vi "Zyklussteuerung.vi"(0 "FPGA VI Reference In":refnum<k20>, 1 "DIOsNummern":cluster{"DIOsMod2BNr":i32[]}[](array[cluster]), 2 "Zyklusnummern 0, 1, 2A, 2B":i32[](array[numeric]), 3 "Zykluszeiten 0, 1, 2A, 2B":dbl[](array[numeric]), 4 "Zeitpkte/SPs":T1 {"FPGAPID"."proportional gain (Kc)" format="%.11g"; "FPGAPID"."integral gain (Kc*Ts/Ti)" format="%.11g"; "FPGAPID"."derivative gain (Kc*Td/Ts)" format="%.11g"; "FPGAFixp" format="%.14g"}, 5 "HorstSP":dbl[](array[numeric]), 6 "ZwangsDIO?":cluster{bool[]}[](array[cluster]), 7 "ZwangsLangsameH?":bool[](array[boolean]), 8 "ZwangsDIO!":cluster{bool[]}[](array[cluster]), 9 "ZwangsLangsameH!":bool[](array[boolean]), 10 "ZwangsHorst?":cluster{bool[]}[](array[cluster]), 11 "ZwangsFPGABoolesch?":bool[](array[boolean]), 12 "ZwangsHorst!":cluster{dbl[]}[](array[cluster]), 13 "ZwangsFPGABoolesch!":bool[](array[boolean]), 14 "Schieberegister":T2) -> (15 "HorstSP":dbl[](array[numeric]), 17 "Heizen?LH":bool[](array[boolean]), 19 "Schieberegister":T2)   [LabVIEW 2010]
uses:
  <vilib>/rvi/interface/nirviReadWriteControl/nirviReadWriteControl.xnode
  C:/Users/HAGAR-IV/Desktop/Zeugs/markus/version feb 2012/FPGA Bitfiles/pertrasgcfpga2_FPGATarget_FPGA-Programm-10_16368CB6.lvbitx
  C:/Users/HAGAR-IV/Desktop/Zeugs/Johnny/pertrasgc fpga/FPGA-Programm-10-14.vi
  <vilib>/rvi/interface/common/niFpgaNodeNameForErrorReporting.ctl
  <vilib>/rvi/errors/niLvFpgaWhatHappensToTopLevelVI.ctl
  <vilib>/Utility/error.llb/Error Cluster From Error Code.vi
  <vilib>/rvi/errors/niLvFpgaAdjustHostInterfaceError.vi
  NiFpgaLv.dll
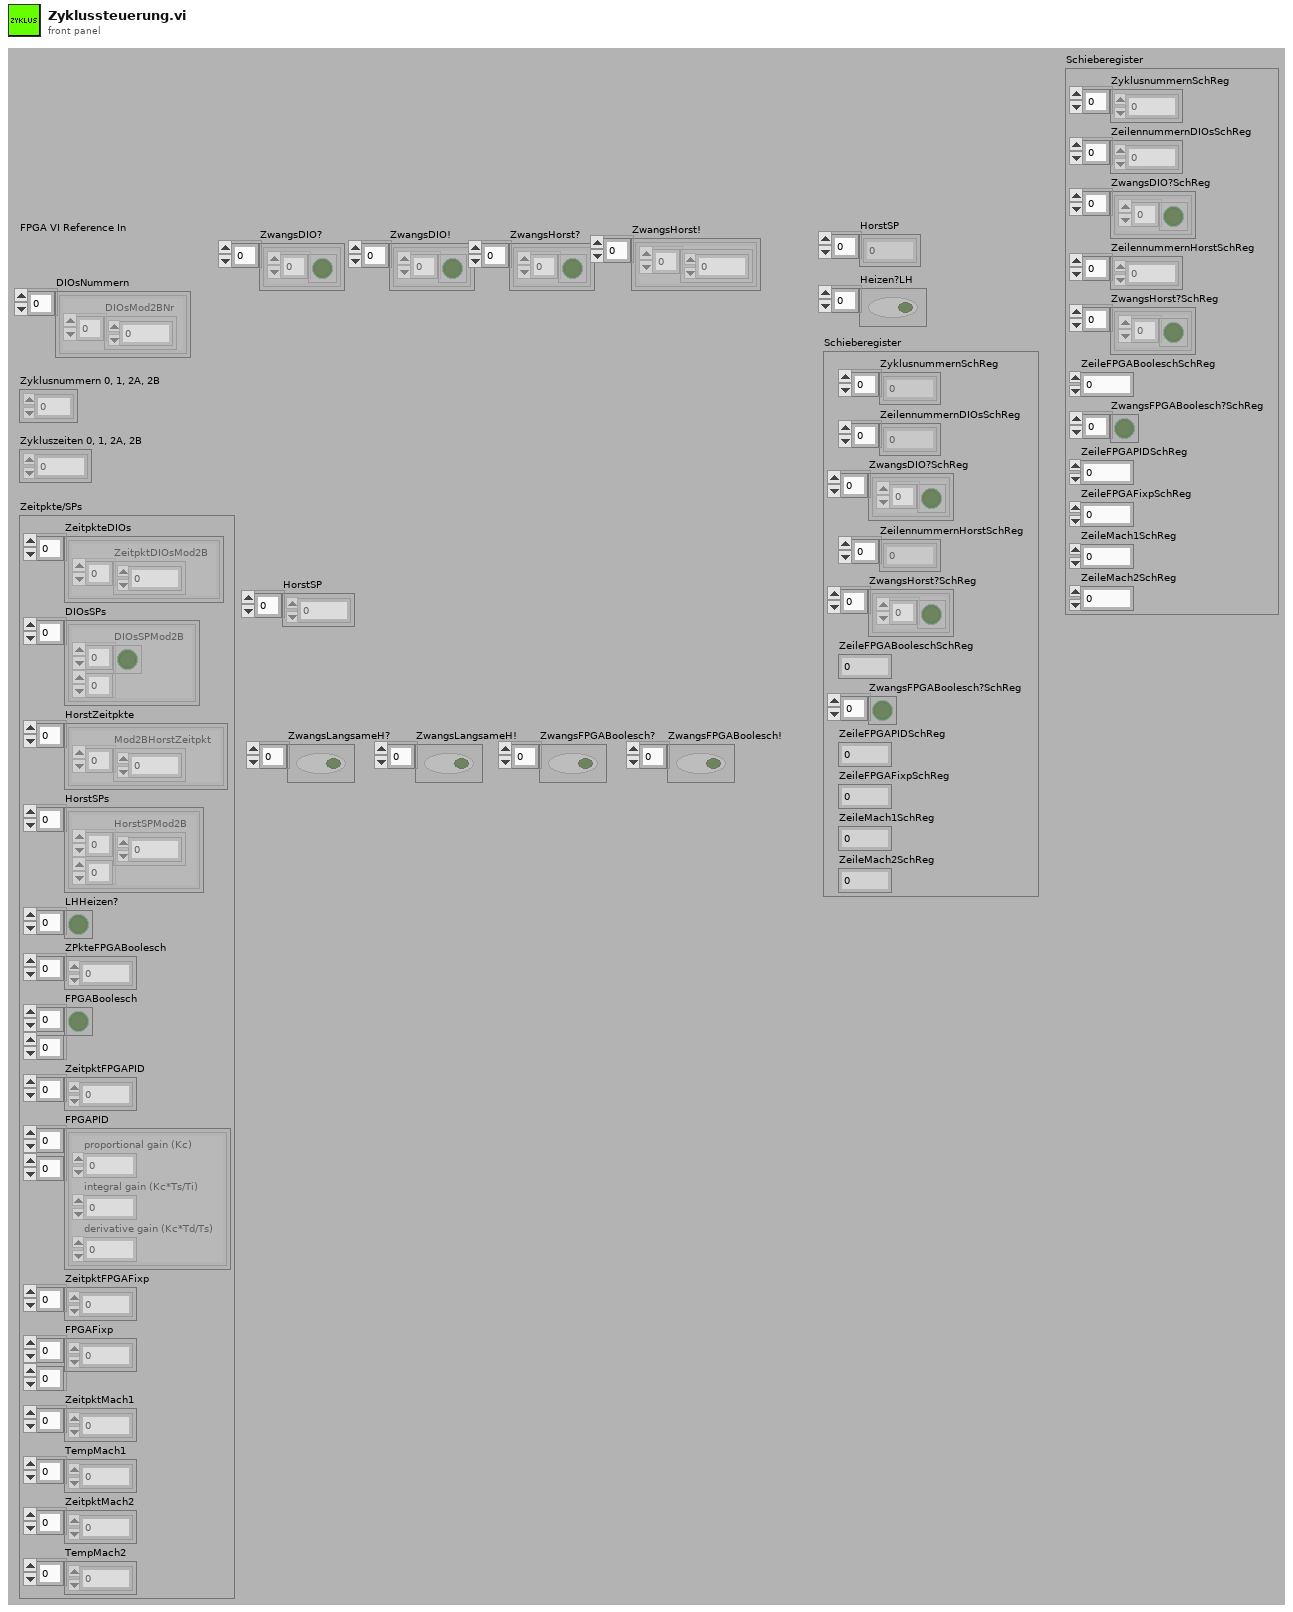
[diagram p1: front panel]
types:
  T1 = cluster{"ZeitpkteDIOs":cluster{"ZeitpktDIOsMod2B":dbl[]}[], "DIOsSPs":cluster{"DIOsSPMod2B":bool[][]}[], "HorstZeitpkte":cluster{"Mod2BHorstZeitpkt":dbl[]}[], "HorstSPs":cluster{"HorstSPMod2B":dbl[][]}[], "LHHeizen?":bool[], "ZPkteFPGABoolesch":dbl[], "FPGABoolesch":bool[][], "ZeitpktFPGAPID":dbl[], "FPGAPID":cluster{"proportional gain (Kc)":fxp<+/-,16,8>, "integral gain (Kc*Ts/Ti)":fxp<+/-,16,8>, "derivative gain (Kc*Td/Ts)":fxp<+/-,16,8>}[][], "ZeitpktFPGAFixp":dbl[], "FPGAFixp":fxp<+/-,16,4>[][], "ZeitpktMach1":dbl[], "TempMach1":dbl[], "ZeitpktMach2":dbl[], "TempMach2":dbl[]}
  T2 = cluster{"ZyklusnummernSchReg":i32[], "ZeilennummernDIOsSchReg":i32[], "ZwangsDIO?SchReg":cluster{bool[]}[], "ZeilennummernHorstSchReg":i32[], "ZwangsHorst?SchReg":cluster{bool[]}[], "ZeileFPGABooleschSchReg":i32, "ZwangsFPGABoolesch?SchReg":bool[], "ZeileFPGAPIDSchReg":i32, "ZeileFPGAFixpSchReg":i32, "ZeileMach1SchReg":i32, "ZeileMach2SchReg":i32}
  T3 = cluster{"proportional gain (Kc)":fxp<+/-,16,8>, "integral gain (Kc*Ts/Ti)":fxp<+/-,16,8>, "derivative gain (Kc*Td/Ts)":fxp<+/-,16,8>}[][]
  T4 = typedef "niFpgaNodeNameForErrorReporting.ctl" = enum16{"Open FPGA VI Reference", "Read/Write Control", "Invoke Method: Abort", "Invoke Method: Acknowledge IRQ", "Invoke Method: Download", "Invoke Method: FIFO.Configure", "Invoke Method: FIFO.Read", "Invoke Method: FIFO.Start", "Invoke Method: FIFO.Stop", "Invoke Method: FIFO.Write", "Invoke Method: Reset", "Invoke Method: Run", "Invoke Method: Wait on IRQ", "Close FPGA VI Reference"}
  T5 = typedef "niLvFpgaWhatHappensToTopLevelVI.ctl" = enum16{"top level VI scripted behind XNode", "top level VI inlined behind XNode"}
  T6 = cluster{"FPGAFixp[0]":fxp<+/-,16,4>, "FPGAFixp[1]":fxp<+/-,16,4>, "FPGAFixp[2]":fxp<+/-,16,4>, "FPGAFixp[3]":fxp<+/-,16,4>, "FPGAFixp[4]":fxp<+/-,16,4>, "FPGAFixp[5]":fxp<+/-,16,4>, "FPGAFixp[6]":fxp<+/-,16,4>, "FPGAFixp[7]":fxp<+/-,16,4>}
  T7 = cluster{"proportional gain (Kc)":fxp<+/-,16,8>, "integral gain (Kc*Ts/Ti)":fxp<+/-,16,8>, "derivative gain (Kc*Td/Ts)":fxp<+/-,16,8>}[]
  T8 = cluster{"FPGAPID[0]":cluster{"proportional gain (Kc)":fxp<+/-,16,8>, "integral gain (Kc*Ts/Ti)":fxp<+/-,16,8>, "derivative gain (Kc*Td/Ts)":fxp<+/-,16,8>}, "FPGAPID[1]":cluster{"proportional gain (Kc)":fxp<+/-,16,8>, "integral gain (Kc*Ts/Ti)":fxp<+/-,16,8>, "derivative gain (Kc*Td/Ts)":fxp<+/-,16,8>}, "FPGAPID[2]":cluster{"proportional gain (Kc)":fxp<+/-,16,8>, "integral gain (Kc*Ts/Ti)":fxp<+/-,16,8>, "derivative gain (Kc*Td/Ts)":fxp<+/-,16,8>}, "FPGAPID[3]":cluster{"proportional gain (Kc)":fxp<+/-,16,8>, "integral gain (Kc*Ts/Ti)":fxp<+/-,16,8>, "derivative gain (Kc*Td/Ts)":fxp<+/-,16,8>}}
  T9 = cluster{"proportional gain (Kc)":fxp<+/-,16,8>, "integral gain (Kc*Ts/Ti)":fxp<+/-,16,8>, "derivative gain (Kc*Td/Ts)":fxp<+/-,16,8>}
  T10 = cluster{"[0]":bool, "[1]":bool, "[2]":bool, "[3]":bool, "[4]":bool, "[5]":bool}
  T11 = cluster{"[0]":bool, "[1]":bool, "[2]":bool, "[3]":bool, "[4]":bool, "[5]":bool, "[6]":bool, "[7]":bool, "[8]":bool, "[9]":bool, "[10]":bool, "[11]":bool, "[12]":bool, "[13]":bool, "[14]":bool, "[15]":bool, "[16]":bool, "[17]":bool, "[18]":bool, "[19]":bool, "[20]":bool, "[21]":bool, "[22]":bool, "[23]":bool, "[24]":bool, "[25]":bool, "[26]":bool, "[27]":bool, "[28]":bool, "[29]":bool, "[30]":bool, "[31]":bool}
  T12 = cluster{"Zyklusnummern 0, 1, 2A, 2B":i32[], i32[], "ZwangsDIO?":cluster{bool[]}[], i32[], "ZwangsHorst?":cluster{bool[]}[], i32, "ZwangsFPGABoolesch?":bool[], i32, i32, i32, i32}
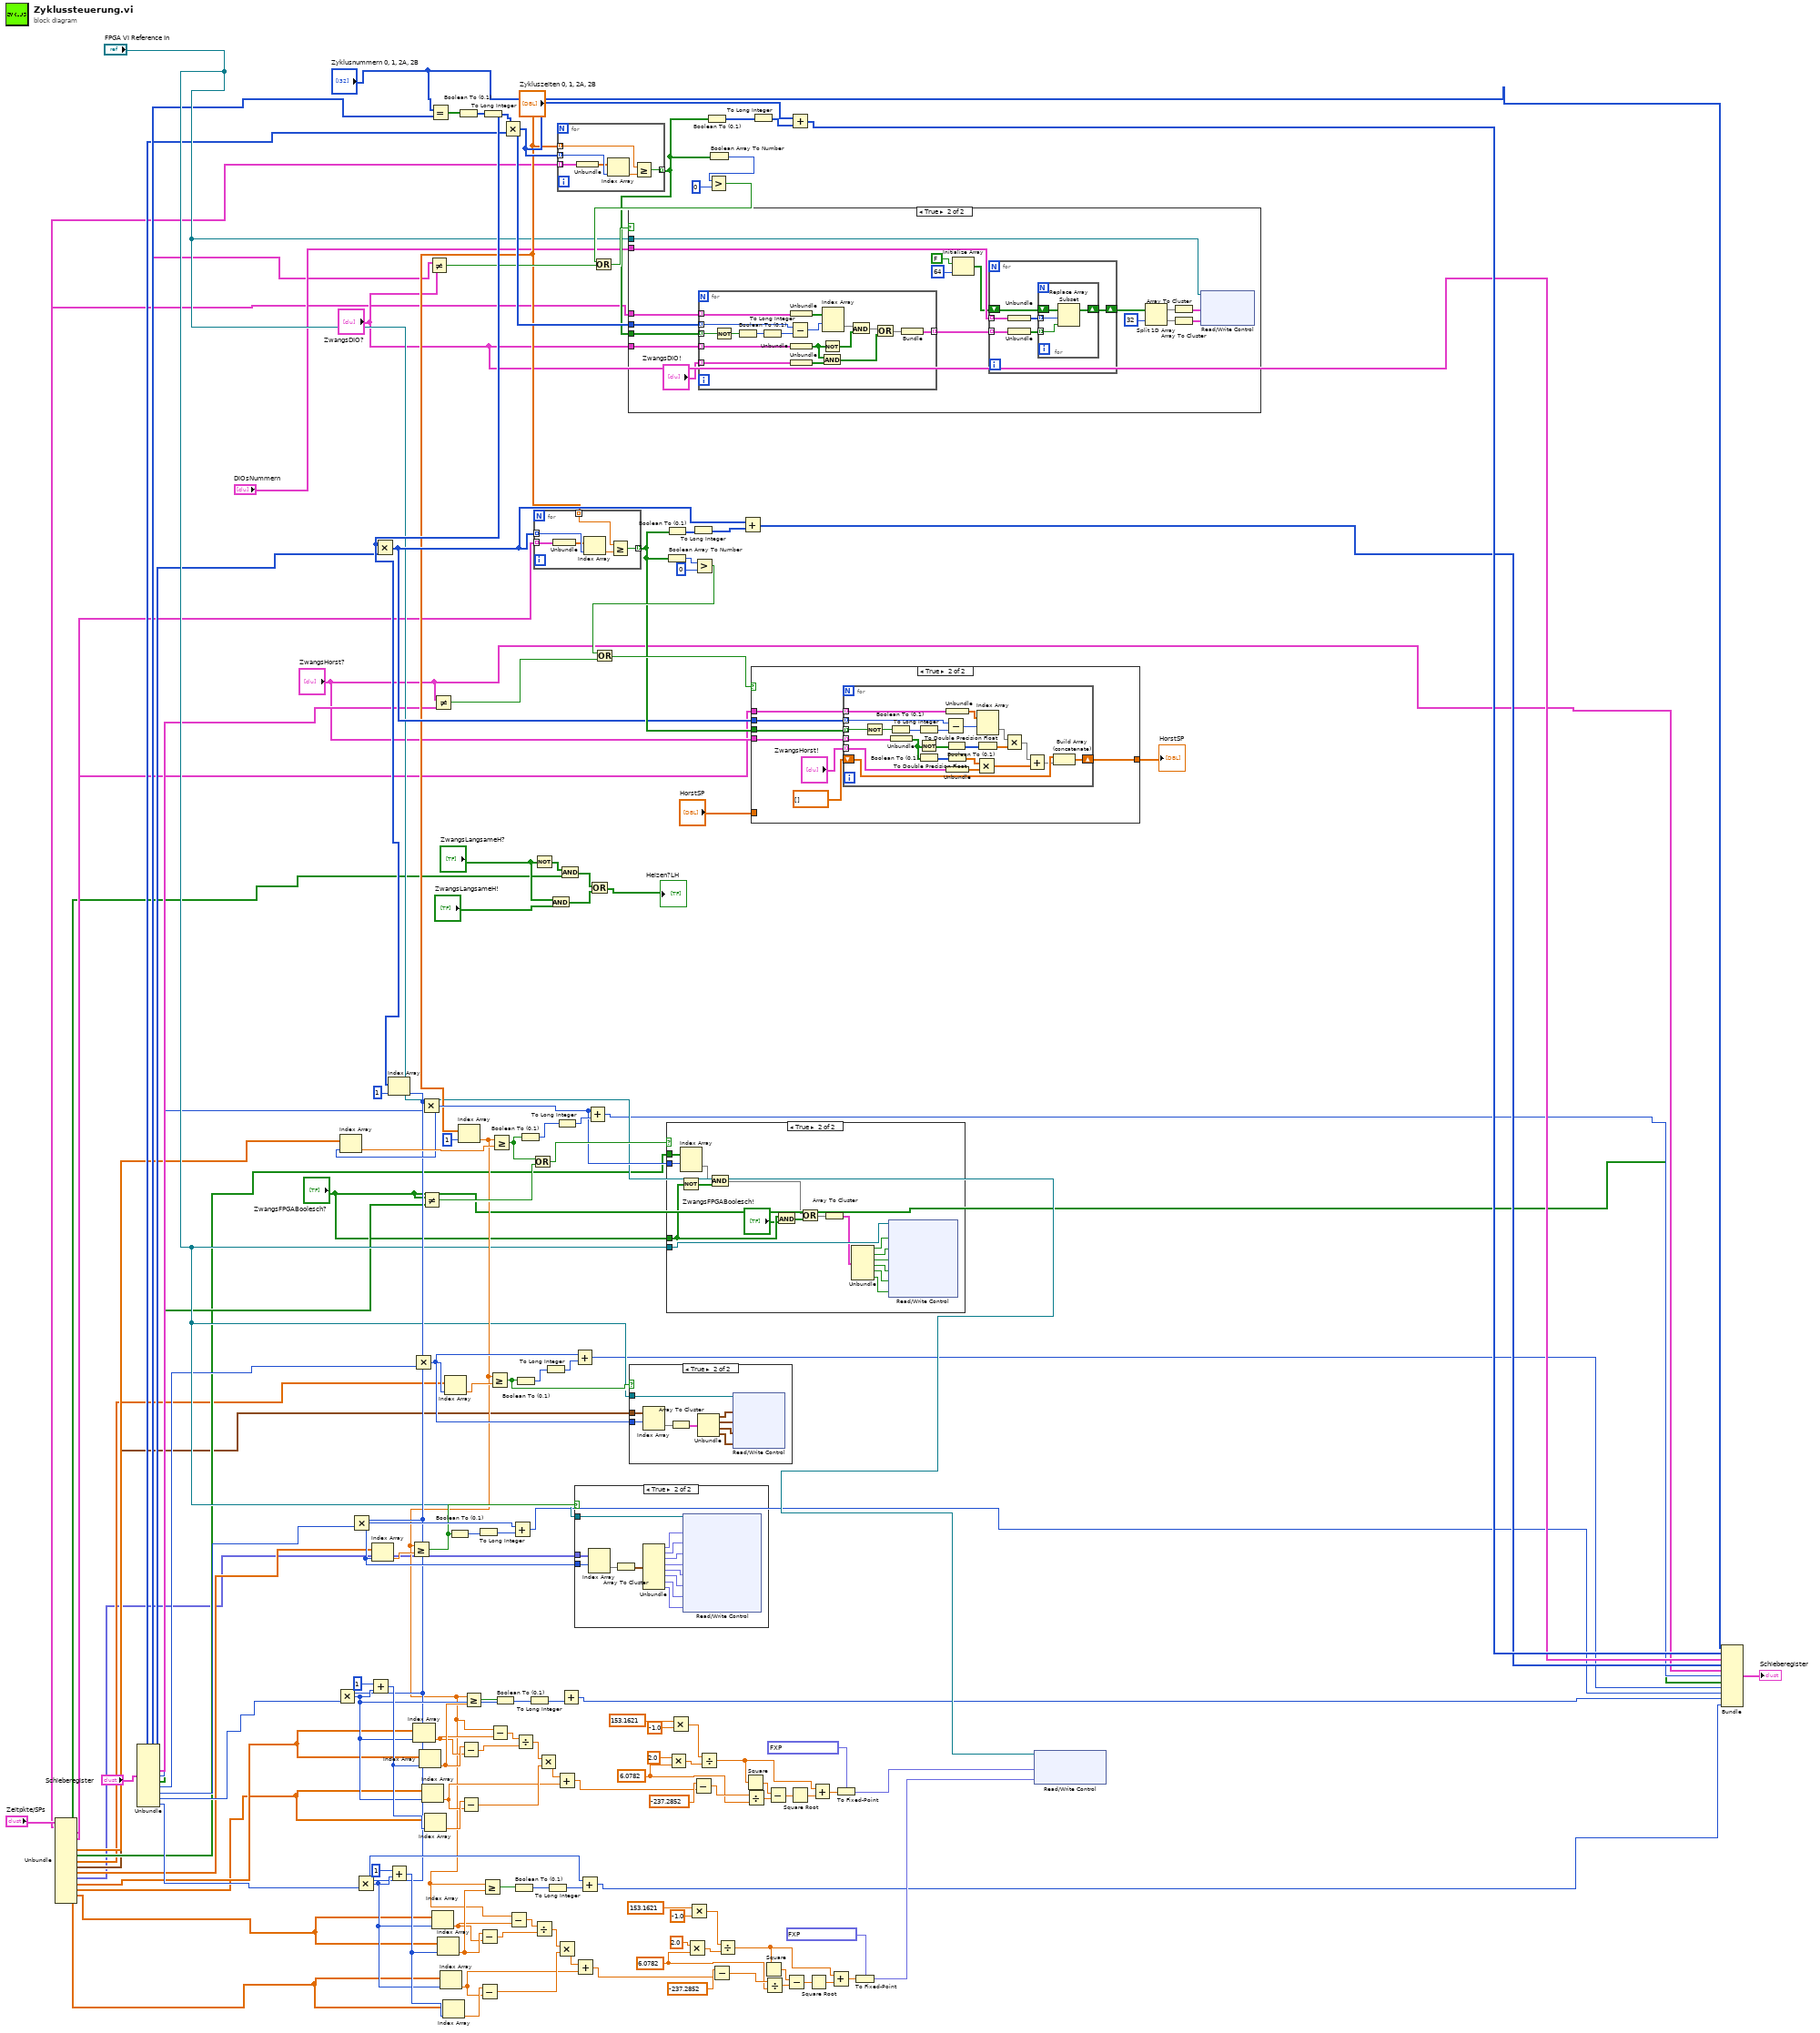
[diagram p0: block diagram]
diagram:
  w67 = 6.0782 ("y")
  w99 = 6.0782 ("y")
  n1 = Unbundle("Zeitpkte/SPs") -> ("ZeitpkteDIOs"=w17:cluster{"ZeitpktDIOsMod2B":dbl[]}[], "DIOsSPs"=w16:cluster{"DIOsSPMod2B":bool[][]}[], "HorstZeitpkte"=w15:cluster{"Mod2BHorstZeitpkt":dbl[]}[], "HorstSPs"=w14:cluster{"HorstSPMod2B":dbl[][]}[], "LHHeizen?"=w13:bool[], "ZPkteFPGABoolesch"=w12:dbl[], "FPGABoolesch"=w11:bool[][], "ZeitpktFPGAPID"=w10:dbl[], "FPGAPID"=w9:T3, "ZeitpktFPGAFixp"=w8:dbl[], "FPGAFixp"=w7:fxp<+/-,16,4>[][], "ZeitpktMach1"=w6:dbl[], "TempMach1"=w5:dbl[], "ZeitpktMach2"=w4:dbl[], "TempMach2"=w3:dbl[])
  n2 = Unbundle("Schieberegister") -> ("ZyklusnummernSchReg"=w41:i32[], "ZeilennummernDIOsSchReg"=w40:i32[], "ZwangsDIO?SchReg"=w39:cluster{bool[]}[], "ZeilennummernHorstSchReg"=w38:i32[], "ZwangsHorst?SchReg"=w37:cluster{bool[]}[], "ZeileFPGABooleschSchReg"=w36:i32, "ZwangsFPGABoolesch?SchReg"=w35:bool[], "ZeileFPGAPIDSchReg"=w34:i32, "ZeileFPGAFixpSchReg"=w33:i32, "ZeileMach1SchReg"=w32:i32, "ZeileMach2SchReg"=w31:i32)
  n3 = Not Equal?(x="ZwangsFPGABoolesch?", y=w35) -> (x != y?=w137:bool)
  n4 = Not Equal?(x=w39, y="ZwangsDIO?") -> (x != y?=w51:bool)
  n5 = Equal?(x="Zyklusnummern 0, 1, 2A, 2B", y=w41) -> (x = y?=w157:bool[])
  n6 = Not Equal?(x="ZwangsHorst?", y=w37) -> (x != y?=w52:bool)
  n7 = Boolean To (0,1)(Boolean=w157) -> (0, 1=w156:i16[])
  n8 = Index Array(array="Zykluszeiten 0, 1, 2A, 2B", index=1 ("Index")) -> (element=w63:dbl)
  n9 = To Long Integer(number=w156) -> (32bit integer=w144:i32[])
  n10 = Multiply(x=w144, y=w38) -> (x*y=w53:i32[])
  n11 = Index Array(array=w144, index=1 ("Index")) -> (element=w64:i32)
  n12 = Multiply(x=w64, y=w32) -> (x*y=w117:i32)
  n13 = Multiply(x=w64, y=w33) -> (x*y=w126:i32)
  n14 = Multiply(x=w64, y=w31) -> (x*y=w87:i32)
  n15 = Add(x=1 ("y"), y=w117) -> (x+y=w123:i32)
  n16 = Index Array(array=w8, index=w126) -> (element=w129:dbl)
  n17 = Add(x=1 ("y"), y=w87) -> (x+y=w93:i32)
  n18 = Greater Or Equal?(x=w63, y=w129) -> (x >= y?=w125:bool)
  n19 = Multiply(x=w64, y=w34) -> (x*y=w130:i32)
  n20 = Index Array(array=w6, index=w117) -> (element=w116:dbl)
  n21 = Index Array(array=w6, index=w123) -> (element=w121:dbl)
  n22 = Multiply(x=w64, y=w36) -> (x*y=w135:i32)
  n23 = Index Array(array=w12, index=w135) -> (element=w141:dbl)
  n24 = Index Array(array=w5, index=w117) -> (element=w110:dbl)
  n25 = Index Array(array=w5, index=w123) -> (element=w122:dbl)
  n26 = Index Array(array=w4, index=w87) -> (element=w86:dbl)
  n27 = Index Array(array=w4, index=w93) -> (element=w91:dbl)
  n28 = Index Array(array=w3, index=w87) -> (element=w80:dbl)
  n29 = Index Array(array=w3, index=w93) -> (element=w92:dbl)
  n30 = Index Array(array=w10, index=w130) -> (element=w134:dbl)
  n31 = Boolean To (0,1)(Boolean=w125) -> (0, 1=w128:i16)
  n32 = Subtract(x=w121, y=w116) -> (x-y=w114:dbl)
  n33 = Subtract(x=w122, y=w110) -> (x-y=w112:dbl)
  n34 = Greater Or Equal?(x=w63, y=w121) -> (x >= y?=w120:bool)
  n35 = To Long Integer(number=w128) -> (32bit integer=w127:i32)
  n36 = Subtract(x=w91, y=w86) -> (x-y=w84:dbl)
  n37 = Subtract(x=w92, y=w80) -> (x-y=w82:dbl)
  n38 = Greater Or Equal?(x=w63, y=w91) -> (x >= y?=w90:bool)
  n39 = Greater Or Equal?(x=w63, y=w134) -> (x >= y?=w131:bool)
  n40 = Subtract(x=w63, y=w116) -> (x-y=w115:dbl)
  n41 = Greater Or Equal?(x=w63, y=w141) -> (x >= y?=w138:bool)
  n42 = Boolean To (0,1)(Boolean=w120) -> (0, 1=w119:i16)
  n43 = Multiply(x=w144, y=w40) -> (x*y=w56:i32[])
  n44 = Subtract(x=w63, y=w86) -> (x-y=w85:dbl)
  n45 = Add(x=w126, y=w127) -> (x+y=w21:i32)
  n46 = Boolean To (0,1)(Boolean=w90) -> (0, 1=w89:i16)
  n47 = Boolean To (0,1)(Boolean=w131) -> (0, 1=w133:i16)
  n48 = Divide(x=w115, y=w114) -> (x/y=w113:dbl)
  n49 = Boolean To (0,1)(Boolean=w138) -> (0, 1=w140:i16)
  n50 = To Long Integer(number=w119) -> (32bit integer=w118:i32)
  n51 = Or(x=w138, y=w137) -> (x .or. y?=w136:bool)
  n52 = Not(x="ZwangsLangsameH?") -> (.not. x?=w61:bool[])
  n53 = Divide(x=w85, y=w84) -> (x/y=w83:dbl)
  n54 = for {
    tunnel: w53 -> [w163] mode=indexing
    tunnel: "Zykluszeiten 0, 1, 2A, 2B" -> [w162] mode=indexing
    tunnel: w15 -> [w159] mode=indexing
    tunnel: [w160] -> w54 mode=indexing
    n55 = Unbundle(w159) -> ("Mod2BHorstZeitpkt"=w158:dbl[])
    n56 = Index Array(array=w158, index=w163) -> (element=w161:dbl)
    n57 = Greater Or Equal?(x=w162, y=w161) -> (x >= y?=w160:bool)
  }
  n58 = Multiply(x=w113, y=w112) -> (x*y=w111:dbl)
  n59 = To Long Integer(number=w133) -> (32bit integer=w132:i32)
  n60 = To Long Integer(number=w89) -> (32bit integer=w88:i32)
  n61 = And(x="ZwangsLangsameH?", y="ZwangsLangsameH!") -> (x .and. y?=w59:bool[])
  n62 = To Long Integer(number=w140) -> (32bit integer=w139:i32)
  n63 = Add(x=w111, y=w110) -> (x+y=w96:dbl)
  n64 = Multiply(x=w83, y=w82) -> (x*y=w81:dbl)
  n65 = for {
    tunnel: w56 -> [w169] mode=indexing
    tunnel: "Zykluszeiten 0, 1, 2A, 2B" -> [w168] mode=indexing
    tunnel: [w167] -> w50 mode=indexing
    tunnel: w17 -> [w165] mode=indexing
    n66 = Unbundle(w165) -> ("ZeitpktDIOsMod2B"=w164:dbl[])
    n67 = Index Array(array=w164, index=w169) -> (element=w166:dbl)
    n68 = Greater Or Equal?(x=w168, y=w166) -> (x >= y?=w167:bool)
  }
  n69 = And(x=w61, y=w13) -> (x .and. y?=w60:bool[])
  n70 = Add(x=w117, y=w118) -> (x+y=w20:i32)
  n71 = Add(x=w130, y=w132) -> (x+y=w22:i32)
  n72 = case shown="True" w125 {
    tunnel: w126 -> [_ w170]
    tunnel: w7 -> [_ w182]
    tunnel: "FPGA VI Reference In" -> [_ w172]
    frame False {
    }
    frame True {
      n73 = Index Array(array=w182, index (row)=w170) -> (element=w171:fxp<+/-,16,4>[])  [unwired: 1 in]
      n74 = Array To Cluster(array=w171) -> (cluster=w181:T6)
      n75 = Unbundle(w181) -> ("FPGAFixp[0]"=w180:fxp<+/-,16,4>, "FPGAFixp[1]"=w179:fxp<+/-,16,4>, "FPGAFixp[2]"=w178:fxp<+/-,16,4>, "FPGAFixp[3]"=w177:fxp<+/-,16,4>, "FPGAFixp[4]"=w176:fxp<+/-,16,4>, "FPGAFixp[5]"=w175:fxp<+/-,16,4>, "FPGAFixp[6]"=w174:fxp<+/-,16,4>, "FPGAFixp[7]"=w173:fxp<+/-,16,4>)
      n76 = xnode "Read/Write Control"("FPGA VI Reference In"=w172, "UTempSPTrap1"=w180, "UTempMaxTrap1"=w179, "UWidrMaxTrap1"=w178, "UTempSPTrap2"=w177, "UTempMaxTrap2"=w176, "UWidrMaxTrap2"=w175, "Umax[V]Mach1"=w174, "Umax[V]Mach2"=w173) -> ()  [unwired: 1 in, 2 out]
    }
  }
  n77 = Add(x=w81, y=w80) -> (x+y=w65:dbl)
  n78 = Add(x=w87, y=w88) -> (x+y=w19:i32)
  n79 = Add(x=w135, y=w139) -> (x+y=w24:i32)
  n80 = Or(x=w60, y=w59) -> (x .or. y?=→"Heizen?LH":bool[])
  n81 = case shown="True" w131 {
    tunnel: "FPGA VI Reference In" -> [_ w432]
    tunnel: w9 -> [_ w431]
    tunnel: w130 -> [_ w424]
    frame False {
    }
    frame True {
      n82 = Index Array(array=w431, index (row)=w424) -> (element=w430:T7)  [unwired: 1 in]
      n83 = Array To Cluster(array=w430) -> (cluster=w429:T8)
      n84 = Unbundle(w429) -> ("FPGAPID[0]"=w428:T9, "FPGAPID[1]"=w427:T9, "FPGAPID[2]"=w426:T9, "FPGAPID[3]"=w425:T9)
      n85 = xnode "Read/Write Control"("FPGA VI Reference In"=w432, "PIDTrap1"=w428, "PIDTrap2"=w427, "PIDMach1"=w426, "PIDMach2"=w425) -> ()  [unwired: 1 in, 2 out]
    }
  }
  n86 = Boolean To (0,1)(Boolean=w54) -> (0, 1=w149:i16[])
  n87 = Boolean Array To Number(Boolean array=w54) -> (number=w147:u32)
  n88 = case shown="True" w136 {
    tunnel: w135 -> [_ w556]
    tunnel: "ZwangsFPGABoolesch?" -> [_ w566]
    tunnel: w11 -> [_ w570]
    tunnel: "FPGA VI Reference In" -> [_ w563]
    frame False {
    }
    frame True {
      n89 = Not(x=w566) -> (.not. x?=w569:bool[])
      n90 = Index Array(array=w570, index (row)=w556) -> (element=w568:bool[])  [unwired: 1 in]
      n91 = And(x=w568, y=w569) -> (x .and. y?=w567:bool[])
      n92 = And(x=w566, y="ZwangsFPGABoolesch!") -> (x .and. y?=w565:bool[])
      n93 = Or(x=w567, y=w565) -> (x .or. y?=w564:bool[])
      n94 = Array To Cluster(array=w564) -> (cluster=w562:T10)
      n95 = Unbundle(w562) -> ("[0]"=w555:bool, "[1]"=w561:bool, "[2]"=w560:bool, "[3]"=w559:bool, "[4]"=w558:bool, "[5]"=w557:bool)
      n96 = xnode "Read/Write Control"("FPGA VI Reference In"=w563, "ServoTrap1kalt"=w555, "ServoTrap2kalt"=w561, "Heizen?Trap1"=w560, "Heizen?Trap2"=w559, "Heizen?Mach1"=w558, "Heizen?Mach2"=w557) -> ()  [unwired: 1 in, 2 out]
    }
  }
  n97 = Multiply(x=2.0, y=w99) -> (x*y=w107:dbl)
  n98 = Multiply(x=153.1621 ("y"), y=-1.0) -> (x*y=w108:dbl)
  n99 = Multiply(x=2.0 ("y"), y=w67) -> (x*y=w75:dbl)
  n100 = Multiply(x=153.1621 ("y"), y=-1.0) -> (x*y=w77:dbl)
  n101 = To Long Integer(number=w149) -> (32bit integer=w148:i32[])
  n102 = Subtract(x=-237.2852 ("y"), y=w96) -> (x-y=w104:dbl)
  n103 = Greater?(x=w147, y=u32 0) -> (0:w145:bool)
  n104 = Or(x=w145, y=w52) -> (x .or. y?=w55:bool)
  n105 = Divide(x=w108, y=w107) -> (x/y=w101:dbl)
  n106 = Boolean To (0,1)(Boolean=w50) -> (0, 1=w155:i16[])
  n107 = Boolean Array To Number(Boolean array=w50) -> (number=w153:u32)
  n108 = Greater?(x=w153, y=u32 0) -> (0:w150:bool)
  n109 = Or(x=w150, y=w51) -> (x .or. y?=w151:bool)
  n110 = case shown="True" w151 {
    tunnel: w56 -> [_ w726]
    tunnel: "ZwangsDIO?" -> [_ w723]
    tunnel: "DIOsNummern" -> [_ w730]
    tunnel: "FPGA VI Reference In" -> [_ w729]
    tunnel: w16 -> [_ w724]
    tunnel: w50 -> [_ w725]
    frame False {
    }
    frame True {
      n111 = for {
        tunnel: w726 -> [w745] mode=indexing
        tunnel: w725 -> [w744] mode=indexing
        tunnel: w724 -> [w743] mode=indexing
        tunnel: w723 -> [w742] mode=indexing
        tunnel: "ZwangsDIO!" -> [w741] mode=indexing
        tunnel: [w731] -> w722 mode=indexing
        n112 = Not(x=w744) -> (.not. x?=w747:bool)
        n113 = Boolean To (0,1)(Boolean=w747) -> (0, 1=w746:i16)
        n114 = To Long Integer(number=w746) -> (32bit integer=w748:i32)
        n115 = Subtract(x=w745, y=w748) -> (x-y=w739:i32)
        n116 = Unbundle(w743) -> ("DIOsSPMod2B"=w740:bool[][])
        n117 = Unbundle(w742) -> (w736:bool[])
        n118 = Unbundle(w741) -> (w735:bool[])
        n119 = Not(x=w736) -> (.not. x?=w737:bool[])
        n120 = And(x=w736, y=w735) -> (x .and. y?=w733:bool[])
        n121 = Index Array(array=w740, index (row)=w739) -> (element=w738:bool[])  [unwired: 1 in]
        n122 = And(x=w738, y=w737) -> (x .and. y?=w734:bool[])
        n123 = Or(x=w734, y=w733) -> (x .or. y?=w732:bool[])
        n124 = Bundle(w732) -> (w731:cluster{bool[]})  [unwired: 1 in]
      }
      n125 = Initialize Array(FALSE, 64 ("Dimension")) -> (w714:bool[])
      n126 = for {
        tunnel: w722 -> [w823] mode=indexing
        tunnel: w730 -> [w825] mode=indexing
        shift-right: [w826] -> w727
        shift-left: w714 -> [w827]
        n127 = Unbundle(w825) -> ("DIOsMod2BNr"=w824:i32[])
        n128 = Unbundle(w823) -> (w822:bool[])
        n129 = for {
          tunnel: w822 -> [w829] mode=indexing
          tunnel: w824 -> [w830] mode=indexing
          shift-right: [w828] -> w826
          shift-left: w827 -> [w831]
          n130 = Replace Array Subset(array=w831, new element=w829, index=w830) -> (w828:bool[])
        }
      }
      n131 = Split 1D Array(array=w727, index=32 ("Länge")) -> (first subarray=w721:bool[], second subarray=w719:bool[])
      n132 = Array To Cluster(array=w721) -> (cluster=w720:T11)
      n133 = Array To Cluster(array=w719) -> (cluster=w718:T11)
      n134 = xnode "Read/Write Control"("FPGA VI Reference In"=w729, "Mod5/DIO"=w720, "Mod6/DIO"=w718) -> ()  [unwired: 1 in, 2 out]
    }
  }
  n135 = Subtract(x=-237.2852 ("y"), y=w65) -> (x-y=w72:dbl)
  n136 = Divide(x=w77, y=w75) -> (x/y=w69:dbl)
  n137 = Add(x=w53, y=w148) -> (x+y=w26:i32[])
  n138 = Square(x=w101) -> (x^2=w106:dbl)
  n139 = Divide(x=w104, y=w99) -> (x/y=w103:dbl)
  n140 = case shown="True" w55 {
    tunnel: w14 -> [_ w836]
    tunnel: "ZwangsHorst?" -> [_ w837]
    tunnel: w54 -> [_ w839]
    tunnel: w53 -> [_ w838]
    tunnel: [w832 w833] -> w2
    tunnel: "HorstSP" -> [w832 _]
    frame False {
    }
    frame True {
      n141 = for {
        tunnel: w839 -> [w859] mode=indexing
        tunnel: w838 -> [w856] mode=indexing
        tunnel: w837 -> [w862] mode=indexing
        tunnel: w836 -> [w860] mode=indexing
        tunnel: "ZwangsHorst!" -> [w861] mode=indexing
        shift-right: [w840] -> w833
        shift-left: dbl[] [] -> [w842]
        n142 = Not(x=w859) -> (.not. x?=w858:bool)
        n143 = Boolean To (0,1)(Boolean=w858) -> (0, 1=w857:i16)
        n144 = Unbundle(w862) -> (w849:bool[])
        n145 = To Long Integer(number=w857) -> (32bit integer=w855:i32)
        n146 = Not(x=w849) -> (.not. x?=w852:bool[])
        n147 = Boolean To (0,1)(Boolean=w849) -> (0, 1=w850:i16[])
        n148 = Subtract(x=w856, y=w855) -> (x-y=w853:i32)
        n149 = Boolean To (0,1)(Boolean=w852) -> (0, 1=w851:i16[])
        n150 = Unbundle(w860) -> ("HorstSPMod2B"=w854:dbl[][])
        n151 = To Double Precision Float(number=w850) -> (double precision float=w846:dbl[])
        n152 = Unbundle(w861) -> (w845:dbl[])
        n153 = Multiply(x=w846, y=w845) -> (x*y=w843:dbl[])
        n154 = Index Array(array=w854, index (row)=w853) -> (element=w848:dbl[])  [unwired: 1 in]
        n155 = To Double Precision Float(number=w851) -> (double precision float=w847:dbl[])
        n156 = Multiply(x=w848, y=w847) -> (x*y=w844:dbl[])
        n157 = Add(x=w844, y=w843) -> (x+y=w841:dbl[])
        n158 = Build Array (concatenate)(w842, w841) -> (w840:dbl[])
      }
    }
  }
  "HorstSP" <- w2
  n159 = To Long Integer(number=w155) -> (32bit integer=w154:i32[])
  n160 = Square(x=w69) -> (x^2=w74:dbl)
  n161 = Divide(x=w72, y=w67) -> (x/y=w71:dbl)
  n162 = Subtract(x=w106, y=w103) -> (x-y=w102:dbl)
  n163 = Subtract(x=w74, y=w71) -> (x-y=w70:dbl)
  n164 = Add(x=w56, y=w154) -> (x+y=w28:i32[])
  n165 = Square Root(x=w102) -> (sqrt(x)=w100:dbl)
  n166 = Square Root(x=w70) -> (sqrt(x)=w68:dbl)
  n167 = Add(x=w101, y=w100) -> (x+y=w98:dbl)
  n168 = Add(x=w69, y=w68) -> (x+y=w49:dbl)
  n169 = To Fixed-Point(fixed-point type=fxp<+/-,16,4> 0.0 ("USetp [V]Mach1"), number=w98) -> (fixed-point=w95:fxp<+/-,16,4>)
  n170 = To Fixed-Point(fixed-point type=fxp<+/-,16,4> 0.0 ("USetp [V]Mach1"), number=w49) -> (fixed-point=w62:fxp<+/-,16,4>)
  n171 = xnode "Read/Write Control"("FPGA VI Reference In"="FPGA VI Reference In", "USetp[V]Mach1"=w95, "USetp[V]Mach2"=w62) -> ()  [unwired: 1 in, 2 out]
  n172 = Bundle("Zyklusnummern 0, 1, 2A, 2B"="Zyklusnummern 0, 1, 2A, 2B", w28, "ZwangsDIO?"="ZwangsDIO?", w26, "ZwangsHorst?"="ZwangsHorst?", w24, "ZwangsFPGABoolesch?"="ZwangsFPGABoolesch?", w22, w21, w20, w19) -> (→"Schieberegister":T12)  [unwired: 1 in]
